vi "Pockels-Bundle modulation setup values.vi"() -> (3 "Pockels modul. setup cluster":T1 {"Dwell time (us)" format="%#_13g"; "Fill time (us)" format="%#_13g"; "Frame Size" items=["100X100"=100, "128X128"=128, "200X200"=200, "256X256"=256, "512X512"=512, "1024x1024"=1024, "2048x2048"=2048]})   [LabVIEW 2017]
uses:
  Typedefs/Pockels modulation setup cluster.ctl
  Typedefs/Frame Size.ctl
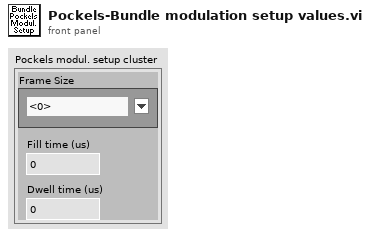
[diagram p1: front panel]
types:
  T1 = typedef "Pockels modulation setup cluster.ctl" = cluster{"Frame Size":T2, "Fill time (us)":dbl, "Dwell time (us)":dbl}
  T2 = typedef "Frame Size.ctl" = u16
  T3 = typedef "AOL_Globals.ctl" = cluster{"Imaging Protocol":T4, "Number of POI":u16, "Number of Miniscans":u16, "Number of Trials":u16, "Number of Cycles ":u64, "# Averaged Frames":u16, "Laser power (%)":u8, "Pockels (V)":dbl, "Acquisition Length (sec)":dbl, "Fill time (us)":dbl, "POI Dwell time (us)":dbl, "Miniscan Dwell time per pixel (us)":dbl, "PMT 1":dbl, "PMT 2":dbl, "Back Apperture (mA)":dbl, "Frame Size":T2, "Center Frequency":dbl, "Field of View (norm)":dbl, "DwellTime (us)":dbl, "Wavelength (nm)":dbl, "Zoom":dbl, "AOL Z":dbl, "AOL Mode":T5, "GridXY":dbl, "GridZ":dbl, "TriggerPeriod (sec)":dbl, "Number of Pixels in Miniscan":u16, "Experiment folder path":path, "X centre":dbl, "Y centre":dbl, "Angle (degrees)":dbl, "Plane Mode":T6, "Threshold":u16[], "Regenerate Chirps":bool, "Rectangle ROI length (pixels)":u16, "Rectangle ROI height (pixels)":u16, "AOD fill":u16, "StartupDelay":i32, "Samples Wait after Trigger":u16, "Slip Cycle":u32, "Add Cycle":bool, "Functional Mode":T7, "Z Start":dbl, "Z Stop":dbl, "# Planes":i32}
  T4 = typedef "Imaging Protocols enum.ctl" = enum16{"AOL Z-Stack", "Motor Z Stack", "Functional Acquisition", "Single Plane Acquisition", "Volume Acquisition", "Live Imaging", "Live Plane Imaging", "Live Volume Imaging"}
  T5 = typedef "AOL modes.ctl" = enum16{"Raster", "Structural", "Pointing", "Mini Scan", "Alignment"}
  T6 = typedef "Plane Mode.ctl" = u16
  T7 = typedef "Functional Mode.ctl" = enum16{"Point", "Line", "Patch", "Plane", "Volume"}
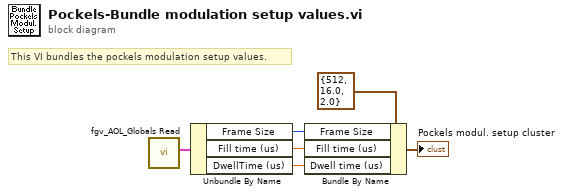
[diagram p0: block diagram]
diagram:
  # "This VI bundles the pockels modulation setup values."
  n1 = call "fgv_AOL_Globals Read.vi"() -> ("AOL_Globals"=w3:T3)  [unwired: 9 in, 2 out]
  n2 = Unbundle By Name(w3) -> ("Frame Size"=w4:T2, "Fill time (us)"=w5:dbl, "DwellTime (us)"=w6:dbl)
  n3 = Bundle By Name(cluster=T1 {"Frame Size"=512, "Fill time (us)"=16.0, "Dwell time (us)"=2.0} ("Input values cluster"), "Frame Size"=w4, "Fill time (us)"=w5, "Dwell time (us)"=w6) -> (→"Pockels modul. setup cluster":T1)
